vi "加载main.vi"(8 "error in (no error)":errorcluster caption="错误输入（无错误）") -> (0 "error out":errorcluster caption="错误输出")   [LabVIEW 2014]
doc: "该模板用于创建子VI。"
uses:
  glb/glb_static.vi
  <vilib>/Utility/config.llb/NI_LVConfig.lvlib
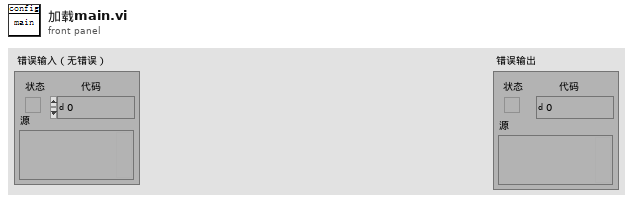
[diagram p1: front panel]
types:
  T1 = typedef "NI_LVConfig.lvlib/Config Data RefNum.ctl" = refnum<k1>
  T2 = cluster{"侧边栏数据":cluster{"来源":string, "名称":string}[], "界面刷间隔率":dbl}
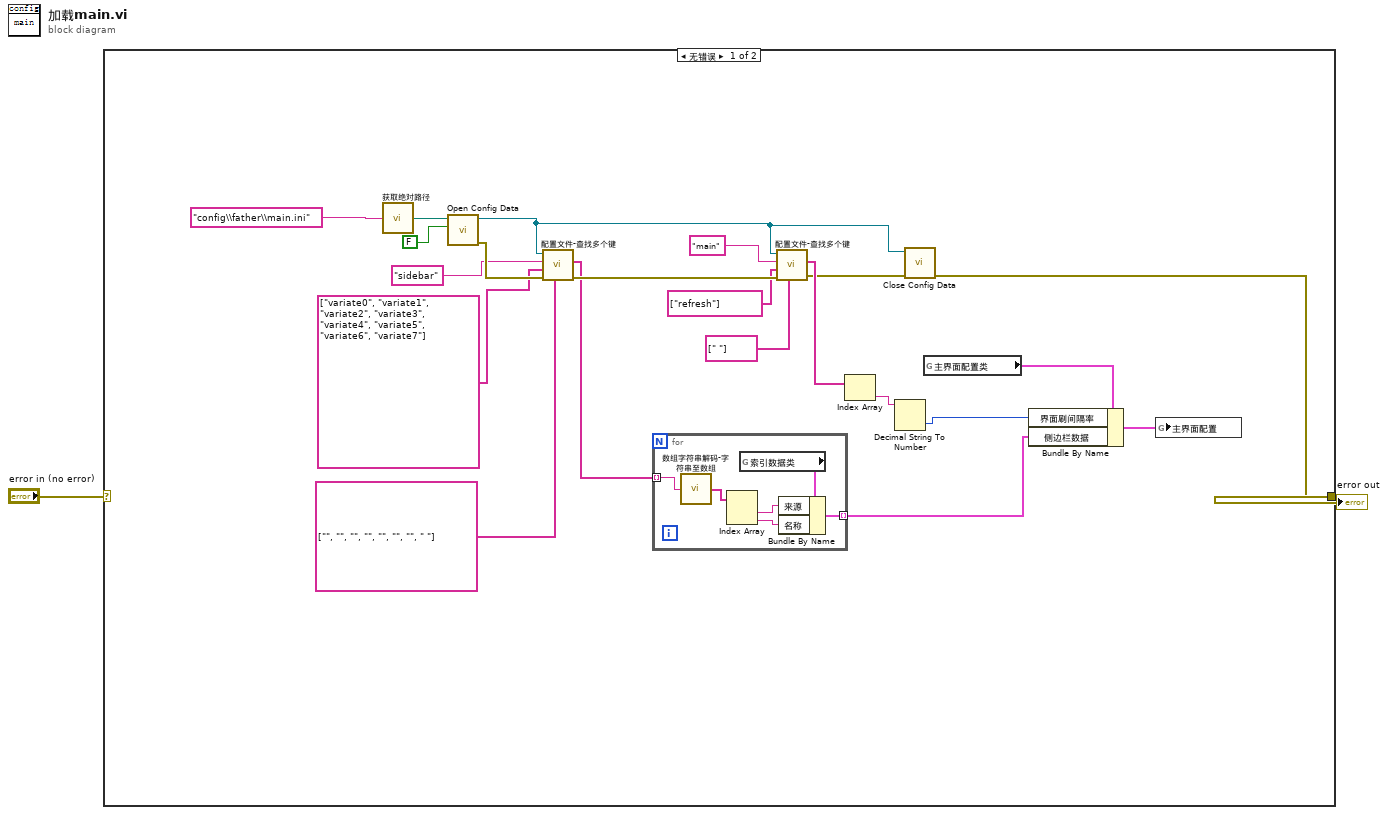
[diagram p0: block diagram]
diagram:
  n1 = case shown="无错误" "error in (no error)" {
    selector: "error in (no error)" -> [_ w30]
    tunnel: [w4 w30] -> w1
    frame No Error {
      n2 = call "获取绝对路径.vi"("relativePath"="config\\father\\main.ini") -> ("absolutePath"=w23:path)
      n3 = call <vilib>:"Open Config Data.vi"("create file if necessary (T)"=FALSE, "configuration file path"=w23) -> ("error out"=w20:errorcluster, "refnum"=w5:T1)  [unwired: 7 in, 1 out]
      n4 = call "配置文件-查找多个键.vi"("默认值"=string[] ["", "", "", "", "", "", "", " "], "错误输入（无错误）"=w20, "键名"=string[] ["variate0", "variate1", "variate2", "variate3", "variate4", "variate5", "variate6", "variate7"], "章名"="sidebar", "引用句柄输入"=w5) -> ("错误输出"=w16:errorcluster, "查询结果"=w12:string[])  [unwired: 4 in, 1 out]
      n5 = for {
        tunnel: w12 -> [w29] mode=indexing
        tunnel: [w24] -> w10 mode=indexing
        n6 = call "数组字符串解码-字符串至数组.vi"("字符串"=w29) -> ("数组"=w27:string[])  [unwired: 1 in]
        n7 = Index Array(array=w27) -> (element #1=w26:string, element #2=w25:string)  [unwired: 2 in]
        n8 = global read "类信息.vi" "索引数据类"() -> (w28:cluster{"来源":string, "名称":string})
        n9 = Bundle By Name(cluster=w28, "来源"=w26, "名称"=w25) -> (w24:cluster{"来源":string, "名称":string})
      }
      n10 = call "配置文件-查找多个键.vi"("默认值"=string[] [" "], "错误输入（无错误）"=w16, "键名"=string[] ["refresh"], "章名"="main", "引用句柄输入"=w5) -> ("错误输出"=w6:errorcluster, "查询结果"=w9:string[])  [unwired: 4 in, 1 out]
      n11 = Index Array(array=w9) -> (element=w8:string)  [unwired: 1 in]
      n12 = Decimal String To Number(string=w8) -> (number=w7:i32)  [unwired: 2 in, 1 out]
      n13 = call <vilib>:"Close Config Data.vi"("error in (no error)"=w6, "refnum"=w5) -> ("error out"=w4:errorcluster)  [unwired: 8 in, 1 out]
      n14 = global read "类信息.vi" "主界面配置类"() -> (w11:T2)
      n15 = Bundle By Name(cluster=w11, "界面刷间隔率"=w7, "侧边栏数据"=w10) -> (w3:T2)
      n16 = global write "glb_static.vi" "主界面配置"(w3) -> ()
    }
    frame Error {
    }
  }
  "error out" <- w1
